vi "Windspeed Warnings.vi"() -> ()   [LabVIEW 2014]
doc: "本VI用于判定基于当前风速值和边界设置的字符串，该字符串输出至气象站。"
uses:
  Weather Data.ctl
panel:
  out "气象数据输出":T1={"当前温度"=0.0, "最高温度"=0.0, "最低温度"=0.0, "温度警告？"=FALSE, "温度警告文本"="无警告", "当前风速"=0.0, "最大风速"=0.0, "风速警告？"=FALSE, "风速警告文本"="无警告"}
  in  "气象数据输入":T1={"当前温度"=0.0, "最高温度"=0.0, "最低温度"=0.0, "温度警告？"=FALSE, "温度警告文本"="无警告", "当前风速"=0.0, "最大风速"=0.0, "风速警告？"=FALSE, "风速警告文本"="无警告"}
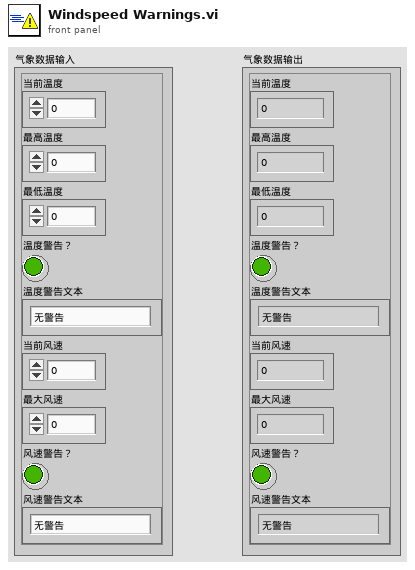
[diagram p1: front panel]
types:
  T1 = typedef "Weather Data.ctl" = cluster{"当前温度":dbl, "最高温度":dbl, "最低温度":dbl, "温度警告？":bool, "温度警告文本":string, "当前风速":dbl, "最大风速":dbl, "风速警告？":bool, "风速警告文本":string}
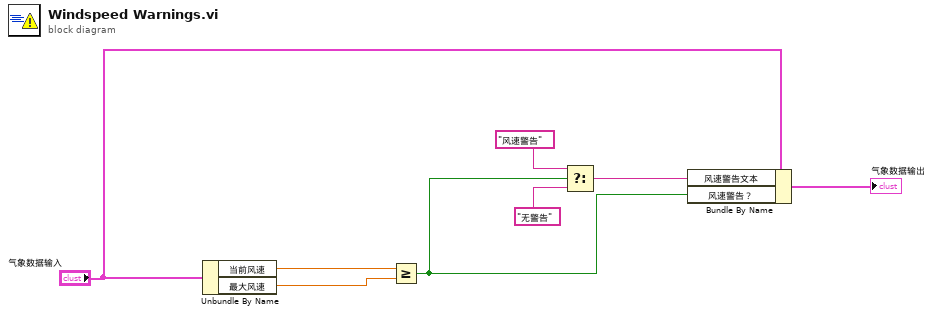
[diagram p0: block diagram]
diagram:
  n1 = Unbundle By Name("气象数据输入") -> ("当前风速"=w8:dbl, "最大风速"=w7:dbl)
  n2 = Greater Or Equal?(x=w8, y=w7) -> (x >= y?=w4:bool)
  n3 = Select(t="风速警告", s=w4, f="无警告") -> (s? t:f=w5:string)
  n4 = Bundle By Name(cluster="气象数据输入", "风速警告文本"=w5, "风速警告？"=w4) -> (→"气象数据输出":T1)
